vi "frontPanel.vi"(8 "error in (no error)":errorcluster, 10 "ScriptEvent":refnum<class "ScriptEvent.lvclass">, 11 "ActionPanel in":refnum<class "Rf_Ramp_Action.lvclass">) -> (0 "error out":errorcluster, 2 "ScriptEvent out":refnum<class "ScriptEvent.lvclass">, 3 "Rf_Ramp_Action out":refnum<class "Rf_Ramp_Action.lvclass">)   [LabVIEW 2009, in "Views.lvlib" / "ScriptEditor.lvlib" / "Rf_Ramp_Action.lvclass"]
uses:
  Rf_Ramp_Action.lvclass
  Tools/Scripting/ScriptingEvent/ScriptEvent.lvclass
  Rf_Ramp_Action.lvclass/Rf_Ramp_Action.ctl
  ActionPanel.lvclass
panel:
  out "ready?":bool
  out "editing":bool
  in  "close":bool
  in  "Number of Steps":dbl format="%#.0f"
  in  "Stop Phase (Degrees)":dbl format="%#.6g"
  in  "Stop Frequency":dbl format="%#.6g"
  in  "Stop Amplitude":string
  in  "Ramp Time":dbl format="%.6g"
  in  "Start Phase (Degrees)":dbl format="%#.6g"
  in  "Start Frequency":dbl format="%#.6g"
  in  "Time":dbl format="%.6g"
  in  "Start Amplitude":string
  in  "Dt":dbl format="%.6g"
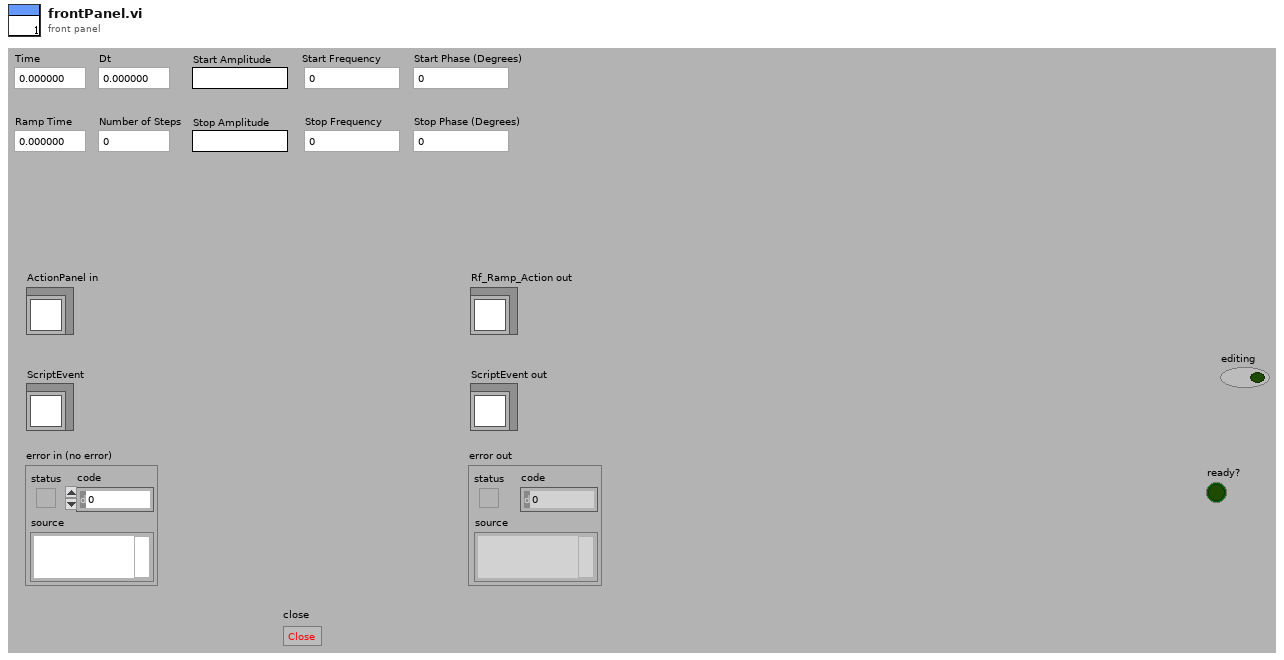
[diagram p1: front panel]
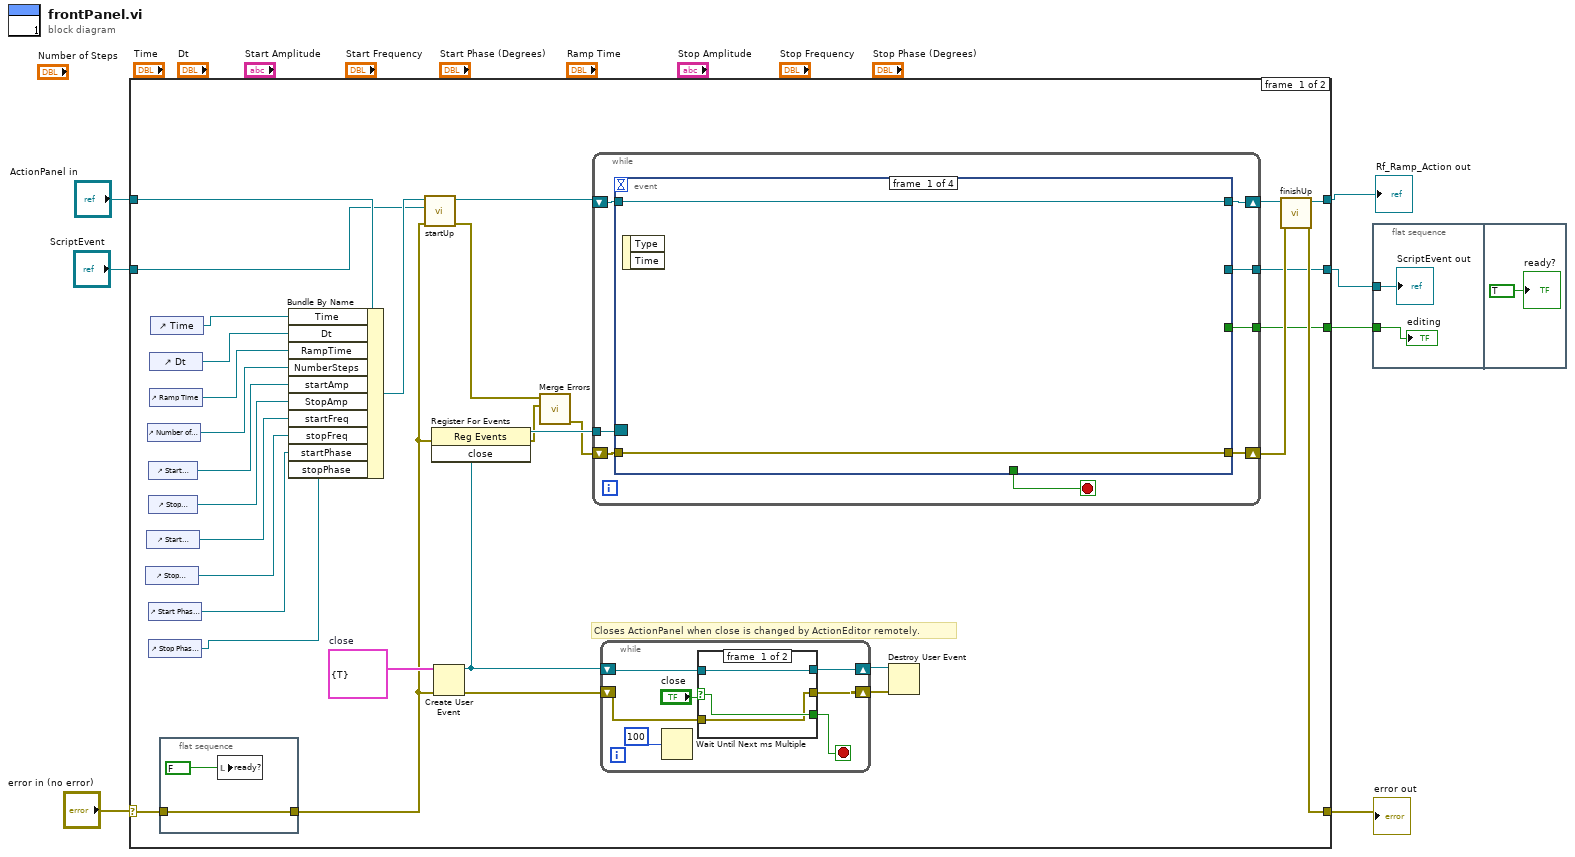
[diagram p0: block diagram]
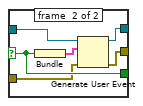
[diagram p2: hidden frame]
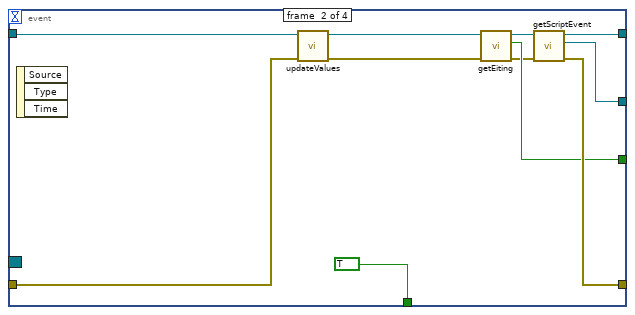
[diagram p3: hidden frame]
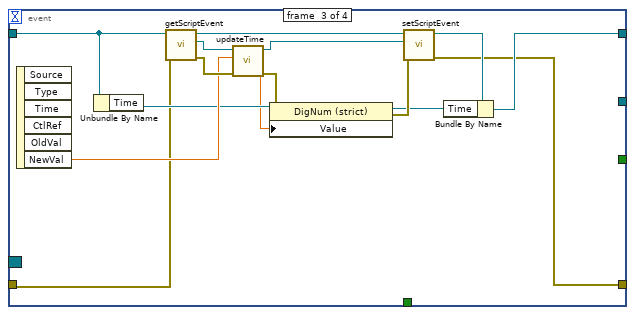
[diagram p4: hidden frame]
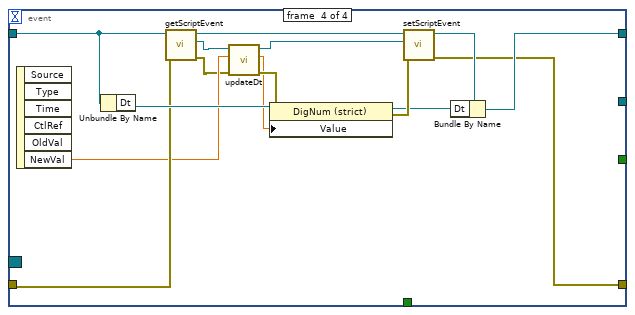
[diagram p5: hidden frame]
diagram:
  n1 = case shown="No Error" "error in (no error)" {
    selector: "error in (no error)" -> [w18 w110]
    tunnel: "ActionPanel in" -> [w38 w109]
    tunnel: "ScriptEvent" -> [w26 w108]
    tunnel: [w10 w110] -> w4
    tunnel: [w12 w109] -> w2
    tunnel: [w9 w108] -> w3
    tunnel: [w8 _] -> w1
    frame #0 {
      w24 = cluster{"close":bool} {"close"=TRUE}  # close
      # "Closes ActionPanel when close is changed by ActionEditor remotely."
      n2 = control-ref of="Stop Frequency"() -> (w35:refnum<vi>)
      n3 = control-ref of="Start Frequency"() -> (w34:refnum<vi>)
      n4 = control-ref of="Number of Steps"() -> (w31:refnum<vi>)
      n5 = control-ref of="Start Amplitude"() -> (w32:refnum<vi>)
      n6 = control-ref of="Stop Amplitude"() -> (w33:refnum<vi>)
      n7 = control-ref of="Start Phase (Degrees)"() -> (w36:refnum<vi>)
      n8 = control-ref of="Stop Phase (Degrees)"() -> (w37:refnum<vi>)
      n9 = control-ref of="Dt"() -> (w29:refnum<vi>)
      n10 = control-ref of="Ramp Time"() -> (w30:refnum<vi>)
      n11 = control-ref of="Time"() -> (w28:refnum<vi>)
      n12 = flat-sequence {
        tunnel: [w39] -> w19
        tunnel: w18 -> [w39]
        frame #0 {
          n13 = local write "ready?"(FALSE) -> ()
        }
      }
      n14 = Bundle By Name(cluster=w38, "Time"=w28, "Dt"=w29, "RampTime"=w30, "NumberSteps"=w31, "startAmp"=w32, "StopAmp"=w33, "startFreq"=w34, "stopFreq"=w35, "startPhase"=w36, "stopPhase"=w37) -> (w27:refnum<class "Rf_Ramp_Action.lvclass">)
      n15 = call-dynamic "startUp.vi"("error in (no error)"=w19, "ScriptEvent"=w26, "Rf_Ramp_Action in"=w27) -> ("error out"=w15:errorcluster, "Rf_Ramp_Action out"=w25:refnum<class "Rf_Ramp_Action.lvclass">)  [unwired: 7 in]
      n16 = Create User Event(user event datatype=w24, error in=w19) -> (user event=w20:refnum<user-event>, error out=w21:errorcluster)
      n17 = register-events(error in=w19, w20) -> (reference out=w17:refnum<event-registration>, error out=w14:errorcluster)  [unwired: 1 in]
      n18 = call <vilib>:"Merge Errors.vi"("error in 2 (no error)"=w14, "error in 1 (no error)"=w15) -> ("error out"=w16:errorcluster)  [unwired: 5 in]
      n19 = while {
        shift-right: [w64] -> w13
        shift-left: w25 -> [w63]
        shift-right: [w59] -> w11
        shift-left: w16 -> [w62]
        tunnel: w17 -> [w60]
        tunnel: [w58] -> w9
        tunnel: [w57] -> w8
        stop <- w61 stop-if-true
        n20 = event shown="[3] \"Time\": Value Change" {
          selector: w60 -> [_ _ _ _]
          dyn-events: _ -> [_ _ _ _]
          timeout: _ -> [_ _ _ _]
          tunnel: [w66 w74 w79 w100] -> w64
          tunnel: w63 -> [w66 w76 w89 w107]
          tunnel: w62 -> [w65 w75 w82 w103]
          tunnel: [_ TRUE _ _] -> w61
          tunnel: [w65 w72 w78 w99] -> w59
          tunnel: [_ w73 _ _] -> w58
          tunnel: [_ w69 _ _] -> w57
          event #0 {
            n21 = event-data() -> ()  [unwired: 1 in, 2 out]
          }
          event #1 {
            n22 = event-data() -> ()  [unwired: 1 in, 3 out]
            n23 = call "updateValues.vi"("error in (no error)"=w75, "Rf_Ramp_Action in"=w76) -> ("error out"=w67:errorcluster, "Rf_Ramp_Action out"=w70:refnum<class "Rf_Ramp_Action.lvclass">)  [unwired: 8 in]
            n24 = call "getEiting.vi"("error in (no error)"=w67, "ActionPanel.lvclass in"=w70) -> ("error out"=w68:errorcluster, "editing?"=w69:bool, "ActionPanel.lvclass out"=w71:refnum<class "Rf_Ramp_Action.lvclass">)  [unwired: 7 in]
            n25 = call "getScriptEvent.vi"("error in (no error)"=w68, "ActionPanel.lvclass in"=w71) -> ("error out"=w72:errorcluster, "ScriptEvent.lvclass"=w73:refnum<class "ScriptEvent.lvclass">, "ActionPanel.lvclass out"=w74:refnum<class "Rf_Ramp_Action.lvclass">)  [unwired: 7 in]
          }
          event #2 {
            n26 = event-data() -> ("NewVal"=w88:dbl)  [unwired: 1 in, 5 out]
            n27 = Unbundle By Name(w89) -> ("Time"=w87:refnum<vi>)
            n28 = call "getScriptEvent.vi"("error in (no error)"=w82, "ActionPanel.lvclass in"=w89) -> ("error out"=w91:errorcluster, "ScriptEvent.lvclass"=w92:refnum<class "ScriptEvent.lvclass">, "ActionPanel.lvclass out"=w81:refnum<class "Rf_Ramp_Action.lvclass">)  [unwired: 7 in]
            n29 = call "updateTime.vi"("error in (no error)"=w91, "time"=w88, "ScriptEvent in"=w92) -> ("error out"=w83:errorcluster, "dt"=w86:dbl, "ScriptEvent out"=w90:refnum<class "ScriptEvent.lvclass">)  [unwired: 6 in]
            n30 = property class="DigNum (strict)"(reference=w87, error in=w83, "Value"=w86) -> (reference out=w80:refnum<vi>, error out=w84:errorcluster)
            n31 = call "setScriptEvent.vi"("error in (no error)"=w84, "ScriptEvent.lvclass"=w90, "ActionPanel.lvclass in"=w81) -> ("error out"=w78:errorcluster, "ActionPanel.lvclass out"=w85:refnum<class "Rf_Ramp_Action.lvclass">)  [unwired: 7 in]
            n32 = Bundle By Name(cluster=w85, "Time"=w80) -> (w79:refnum<class "Rf_Ramp_Action.lvclass">)
          }
          event #3 {
            n33 = event-data() -> ("NewVal"=w96:dbl)  [unwired: 1 in, 5 out]
            n34 = Unbundle By Name(w107) -> ("Dt"=w106:refnum<vi>)
            n35 = call "getScriptEvent.vi"("error in (no error)"=w103, "ActionPanel.lvclass in"=w107) -> ("error out"=w95:errorcluster, "ScriptEvent.lvclass"=w98:refnum<class "ScriptEvent.lvclass">, "ActionPanel.lvclass out"=w102:refnum<class "Rf_Ramp_Action.lvclass">)  [unwired: 7 in]
            n36 = call "updateDt.vi"("error in (no error)"=w95, "dt"=w96, "ScriptEvent in"=w98) -> ("error out"=w94:errorcluster, "time"=w93:dbl, "ScriptEvent out"=w97:refnum<class "ScriptEvent.lvclass">)  [unwired: 6 in]
            n37 = property class="DigNum (strict)"(reference=w106, error in=w94, "Value"=w93) -> (reference out=w101:refnum<vi>, error out=w104:errorcluster)
            n38 = call "setScriptEvent.vi"("error in (no error)"=w104, "ScriptEvent.lvclass"=w97, "ActionPanel.lvclass in"=w102) -> ("error out"=w99:errorcluster, "ActionPanel.lvclass out"=w105:refnum<class "Rf_Ramp_Action.lvclass">)  [unwired: 7 in]
            n39 = Bundle By Name(cluster=w105, "Dt"=w101) -> (w100:refnum<class "Rf_Ramp_Action.lvclass">)
          }
        }
      }
      n40 = while {
        shift-right: [w43] -> w22
        shift-left: w21 -> [w42]
        shift-right: [w44] -> w23
        shift-left: w20 -> [w47]
        stop <- w45 stop-if-true
        n41 = Wait Until Next ms Multiple(millisecond multiple=100) -> ()  [unwired: 1 out]
        n42 = case shown="True" "close" {
          selector: "close" -> [w50 w54]
          tunnel: w47 -> [w49 w56]
          tunnel: [w50 w54] -> w45
          tunnel: [w49 w53] -> w44
          tunnel: [w48 w52] -> w43
          tunnel: w42 -> [w48 w51]
          frame #0 {
          }
          frame #1 {
            n43 = Bundle(w54) -> (w55:cluster{bool})  [unwired: 1 in]
            n44 = Generate User Event(user event=w56, event data cluster=w55, error in=w51) -> (user event out=w53:refnum<user-event>, error out=w52:errorcluster)
          }
        }
      }
      n45 = Destroy User Event(user event=w23, error in=w22) -> ()  [unwired: 1 out]
      n46 = call-dynamic "finishUp.vi"("error in (no error)"=w11, "Rf_Ramp_Action in"=w13) -> ("error out"=w10:errorcluster, "Rf_Ramp_Action out"=w12:refnum<class "Rf_Ramp_Action.lvclass">)  [unwired: 8 in]
    }
    frame #1 {
    }
  }
  "error out" <- w4
  "Rf_Ramp_Action out" <- w2
  n47 = flat-sequence {
    tunnel: w3 -> [w112]
    tunnel: w1 -> [w111]
    frame #0 {
      "editing" <- w111
      "ScriptEvent out" <- w112
    }
    frame #1 {
      "ready?" <- TRUE
    }
  }
